vi "Read.ProcessData.Detect.vi"(4 "length":i32=-1, 6 "index":i32, 8 "error in":errorcluster, 10 "timeout ms":i32, 11 "Read in":refnum<class "Read.lvclass">) -> (0 "error out":errorcluster, 1 "Timeout?":bool, 2 "Data":dbl[](array[numeric]), 3 "Read out":refnum<class "Read.lvclass">, 5 "Detect?":bool[](array[boolean]))   [LabVIEW 2027, in "Data Access Engine (Express).lvlib" / "Read.lvclass"]
uses:
  Read.lvclass
  Read.lvclass/Read.ctl
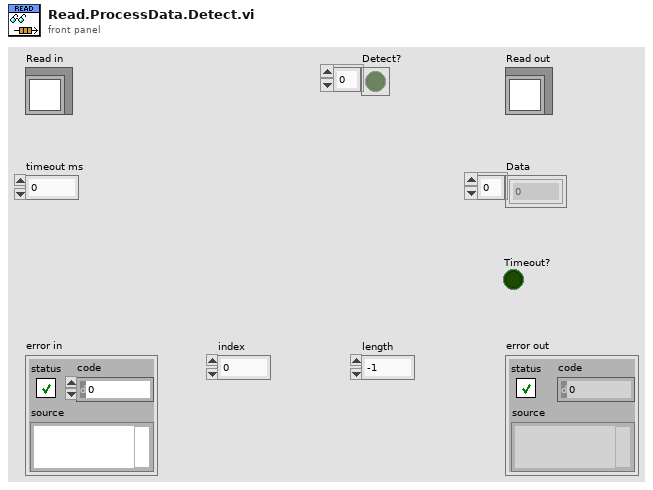
[diagram p1: front panel]
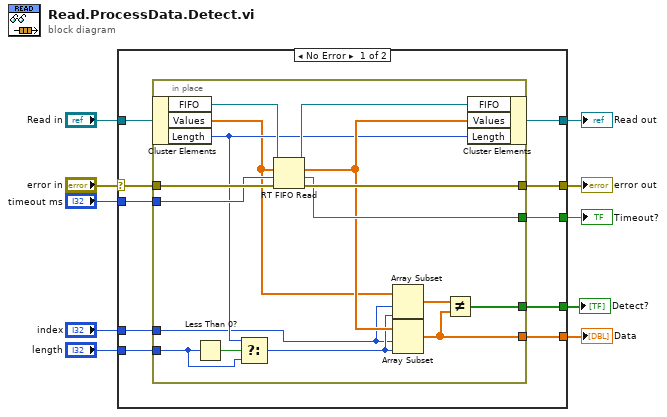
[diagram p0: block diagram]
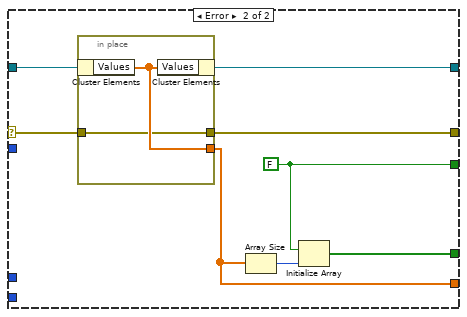
[diagram p2: hidden frame]
diagram:
  n1 = case shown="No Error" "error in" {
    selector: "error in" -> [w18 w44]
    tunnel: [w17 w41] -> w9
    tunnel: [w19 w42] -> w7
    tunnel: "Read in" -> [w20 w43]
    tunnel: "timeout ms" -> [w16 _]
    tunnel: [w15 w40] -> w5
    tunnel: [w14 w38] -> w4
    tunnel: "length" -> [w13 _]
    tunnel: "index" -> [w12 _]
    tunnel: [w11 w37] -> w1
    frame No Error {
      n2 = in-place {
        in-place-border: w18 -> [w34]
        in-place-border: [w33] -> w17
        in-place-border: w16 -> [w32]
        in-place-border: [w23] -> w15
        in-place-border: [w31] -> w14
        in-place-border: w13 -> [w29]
        in-place-border: w12 -> [w24]
        in-place-border: [w21] -> w11
        n3 = in-place-cluster #1(w20) -> ("FIFO"=w36:refnum<k33>, "Values"=w26:dbl[], "Length"=w27:i32)
        n4 = Less Than 0?(x=w29) -> (x < 0?=w30:bool)
        n5 = Select(t=w27, s=w30, f=w29) -> (s? t:f=w25:i32)
        n6 = RT FIFO Read(0:w36, 1:w26, 2:w32, 3:w34) -> (8:w35:refnum<k33>, 9:w28:dbl[], 10:w31:bool, 11:w33:errorcluster)  [unwired: 1 out]
        n7 = Array Subset(array=w26, index=w24, length=w25) -> (w22:dbl[])
        n8 = Array Subset(array=w28, index=w24, length=w25) -> (w23:dbl[])
        n9 = Not Equal?(x=w22, y=w23) -> (x != y?=w21:bool[])
        n10 = in-place-cluster #1("FIFO"=w35, "Values"=w28, "Length"=w27) -> (w19:refnum<class "Read.lvclass">)
      }
    }
    frame Error {
      w38 = FALSE ("empty?")
      n11 = in-place {
        in-place-border: w44 -> [w45]
        in-place-border: [w45] -> w41
        in-place-border: [w46] -> w40
        n12 = in-place-cluster #2(w43) -> ("Values"=w46:dbl[])
        n13 = in-place-cluster #2("Values"=w46) -> (w42:refnum<class "Read.lvclass">)
      }
      n14 = Array Size(array=w40) -> (size(s)=w39:i32)
      n15 = Initialize Array(w38, w39) -> (w37:bool[])
    }
  }
  "error out" <- w9
  "Read out" <- w7
  "Data" <- w5
  "Timeout?" <- w4
  "Detect?" <- w1
